vi "打开相机.vi"(8 "error in":errorcluster, 9 "FPS":u32, 10 "分辨率":string(combo)) -> (0 "error out":errorcluster, 2 "DevCfgGet":cluster{"pid":u32, "vid":u32, "ser_num":u64}[](array[cluster]), 3 "result":bool)   [LabVIEW 2016]
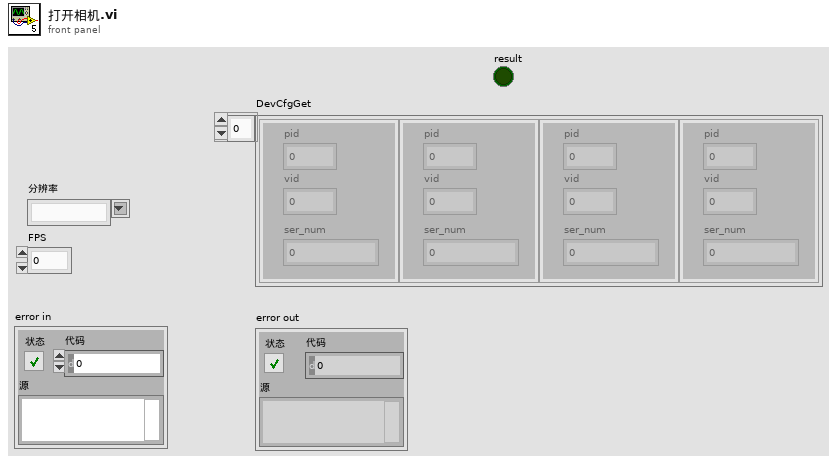
[diagram p1: front panel]
types:
  T1 = cluster{"format":u64, "width":u32, "height":u32, "frame_size":u32, "fps":u32[]}[]
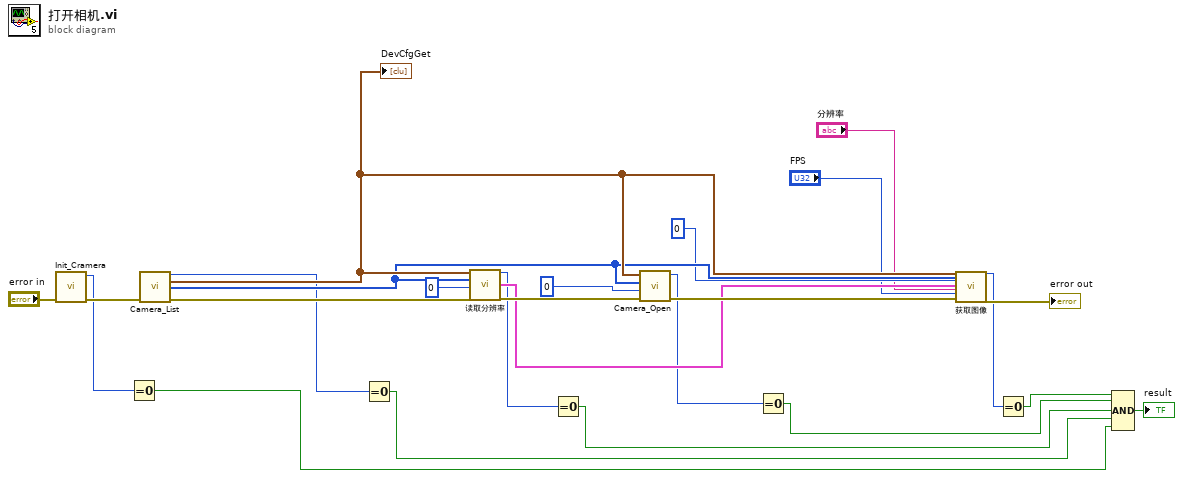
[diagram p0: block diagram]
diagram:
  n1 = call "Init_Cramera.vi"("error in"="error in") -> ("error out"=w25:errorcluster, "初始化返回值"=w7:i32)  [unwired: 9 in]
  n2 = Equal To 0?(x=w7) -> (x = 0?=w2:bool)
  n3 = call "Camera_List.vi"("error in"=w25) -> ("获取设备列表返回值"=w8:i32, "DevCfgGet"=w19:cluster{"pid":u32, "vid":u32, "ser_num":u64}[], "设备列表"=w18:i32[], "error out"=w24:errorcluster)  [unwired: 11 in]
  "DevCfgGet" <- w19
  n4 = Equal To 0?(x=w8) -> (x = 0?=w3:bool)
  n5 = call "读取分辨率.vi"("DevCfgGet"=w19, "设备列表"=w18, "设备"=0, "error in"=w24) -> ("获取设备信息返回值"=w9:i32, "camera_stream_info[]"=w16:T1, "error out"=w22:errorcluster)  [unwired: 9 in]
  n6 = Equal To 0?(x=w9) -> (x = 0?=w4:bool)
  n7 = call "Camera_Open.vi"("error in"=w22, "设备"=0, "设备列表"=w18, "DevCfgGet"=w19) -> ("error out"=w20:errorcluster, "打开设备返回值"=w10:i32)  [unwired: 6 in]
  n8 = Equal To 0?(x=w10) -> (x = 0?=w5:bool)
  n9 = call "获取图像.vi"("DevCfgGet"=w19, "设备列表"=w18, "设备"=0, "camera_stream_info"=w16, "分辨率"="分辨率", "FPS"="FPS", "error in"=w20) -> ("内部出图返回值"=w11:i32, "error out"=→"error out":errorcluster)  [unwired: 19 in]
  n10 = Equal To 0?(x=w11) -> (x = 0?=w6:bool)
  n11 = Compound Arithmetic op=AND(w6, w5, w4, w3, w2) -> (→"result":bool)
